vi "Double Click.vi"(11 "Time":u32) -> (3 "Double Click":bool)   [LabVIEW 2021]
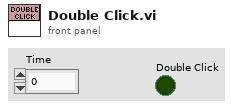
[diagram p1: front panel]
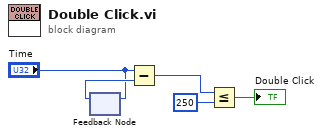
[diagram p0: block diagram]
diagram:
  n1 = feedback #1() -> (w5:u32)  [unwired: 1 in]
  n2 = feedback-in #1("Time") -> ()
  n3 = Subtract(x="Time", y=w5) -> (x-y=w4:u32)
  n4 = Less Or Equal?(x=w4, y=u32 250) -> (x <= y?=→"Double Click":bool)
